vi "Stop Test.vi"(8 "error in (no error)":errorcluster, 11 "Execution Profiler In":refnum<class "Execution Profiler.lvclass">) -> (0 "error out":errorcluster, 3 "Execution Profiler Out":refnum<class "Execution Profiler.lvclass">)   [LabVIEW 2020, in "Execution Profiler.lvlib" / "Execution Profiler.lvclass"]
uses:
  Execution Profiler.lvclass
  Execution Profiler.lvclass/Execution Profiler.ctl
  Execution Profiler View.vi
  Execution Profiler Result View/Execution Profiler Result View.lvclass
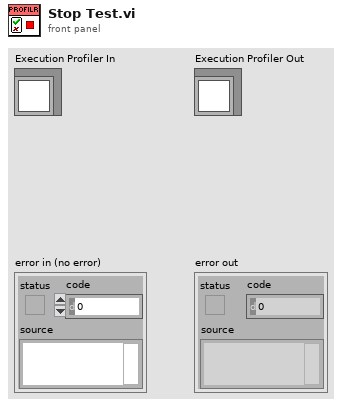
[diagram p1: front panel]
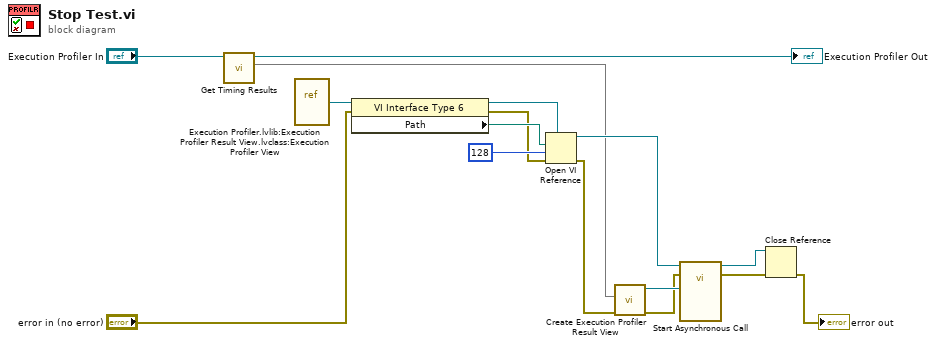
[diagram p0: block diagram]
diagram:
  n1 = call "Get Timing Results.vi"("Execution Profiler in"="Execution Profiler In") -> ("Timing Results"=w1:map{string, dbl}, "Execution Profiler out"=→"Execution Profiler Out":refnum<class "Execution Profiler.lvclass">)  [unwired: 8 in, 1 out]
  n2 = vi-ref "Execution Profiler.lvlib:Execution Profiler Result View.lvclass:Execution Profiler View.vi"() -> (w11:refnum<vi>)
  n3 = property class="VI Interface Type 6"(reference=w11, error in="error in (no error)") -> (reference out=w13:refnum<vi>, error out=w8:errorcluster, "Path"=w12:path)
  n4 = Open VI Reference(type specifier VI Refnum (for type only)=w13, vi path=w12, options=128, error in (no error)=w8) -> (vi reference=w10:refnum<vi>, error out=w4:errorcluster)  [unwired: 2 in]
  n5 = call "Create Execution Profiler Result View.vi"("error in (no error)"=w4, "Timing Results"=w1) -> ("error out"=w3:errorcluster, "Execution Profiler Result View out"=w9:refnum<class "Execution Profiler Result View.lvclass">)  [unwired: 8 in]
  n6 = call-by-ref "Start Asynchronous Call"(reference=w10, error in=w3, "Execution Profiler Result View"=w9) -> (reference out=w16:refnum<vi>, error out=w15:errorcluster)  [unwired: 10 in, 1 out]
  n7 = Close Reference(reference=w16, error in (no error)=w15) -> (error out=→"error out":errorcluster)
